vi "FPGA Main.vi"   [LabVIEW 2021]
uses:
  <vilib>/Platform/TimedLoop/XDataNode/timing_clust.ctl
  <vilib>/Platform/TimedLoop/XDataNode/nitl_modes.ctl
  <vilib>/Platform/TimedLoop/XDataNode/wakeup.ctl
  <vilib>/rvi/Emulation/niFpgaGetClockAttributes.vi
  <vilib>/rvi/Emulation/niFpgaSctlEmulationGetInTimedLoop.vi
  <vilib>/rvi/Emulation/niFpgaEmulationReportErrorSimple.vi
  <vilib>/rvi/DataTransferAndStorage/Container/Common/niFpgaContainerGetUniqueNameForEmu.vi
  <vilib>/rvi/DataTransferAndStorage/Container/Common/niFpgaContainerSetEmuInfo.vi
  <vilib>/rvi/eio/common/nirviEmuReportErrorAndStop.vi
  <vilib>/rvi/interface/RandomDataEmulation/niFpgaRandomDataHandleErrors.vi
  <vilib>/rvi/DataTransferAndStorage/Container/Common/niFpgaContainerExecOnDevCompGetState.vi
  <vilib>/rvi/Emulation/niFpgaEmulationIsFPGAContextNoSignature.vi
  <vilib>/rvi/errors/niFpgaSetErrorForExecOnDevCompSimple.vi
  <vilib>/rvi/FIFO/Fifo_Resource/nirvififoEmulationSetSize.vi
  <vilib>/rvi/FIFO/Fifo_Resource/nirviFifoEmulationQueueMgr.vi
  <instcachedir>/0/nirviFifoEmulationQueueMgr_E5CAEC123FF24DC58D834DCA3CDAA9B5.lvgen/nirviFifoEmulationQueueMgr_E5CAEC123FF24DC58D834DCA3CDAA9B5_002.vi
  <vilib>/rvi/FIFO/Fifo_Resource/nirvififoEmulationDetermineInputValidOut.vi
  <vilib>/rvi/FIFO/Fifo_Resource/nirvififoEmulationCreateLock.vi
  <vilib>/rvi/Emulation/niFpgaProcessEmulError.vi
  <vilib>/rvi/FIFO/Fifo_Resource/nirvififoEmulationObtainLock.vi
  <vilib>/rvi/FIFO/Fifo_Resource/nirvififoEmulationReleaseLock.vi
  <vilib>/rvi/occurrence/nirviWaitOnOccurrenceBase.vi
  <vilib>/rvi/errors/nirviReportUnexpectedCaseInternalError.vi
  <vilib>/rvi/errors/nirviReportUnexpectedCaseInternalError (U32).vi
  <vilib>/Utility/error.llb/Clear Errors.vi
  <vilib>/rvi/Emulation/niFpgaCriticalErrorInLSC.vi
  <vilib>/rvi/eio/common/nirviEmuTemplateMethod_errors.vi
  <vilib>/Platform/TimedLoop/XDataNode/XDataNode.xnode
  <vilib>/rvi/LocalResourceManager/LocalResourceManager.xnode
  <vilib>/rvi/DataTransferAndStorage/Container/XNode/niFpgaContainer.xnode
  <vilib>/rvi/interface/RandomDataEmulation/nirviRandomDataFpgaReadWriteTemplate.vi
  <vilib>/rvi/FIFO/Fifo_Resource/niFpgaFifoEmulationRefIn.vi
  <vilib>/eio/EIONode/EIONode.xnode
  <vilib>/Platform/TimedLoop/XDataNode/XDNodeRunTimeDep.lvlib
types:
  T1 = typedef "XDNodeRunTimeDep.lvlib/timing_clust.ctl" = cluster{"Expected End [f-1]":u64, "Actual End [f-1]":u64, "Finished Late? [f-1]":bool, "Expected End [i-1]":u64, "Actual End [i-1]":u64, "Finished Late? [i-1]":bool, "Expected Start [i]":u64, "Actual Start [i]":u64, "Expected Start [f]":u64, "Actual Start [f]":u64, "Source Name":string, "Structure Name":string, "Period":i64, "Deadline":i64, "Offset":i64, "Start":i64, "Priority":i32, "Timeout":i32, "Mode":T2, "Wakeup Reason":T3, "Error":errorcluster, "Source Type":string, "Secondary Source Type":string, "Global End Time":u64, "Global Start Time":u64, "Frame Duration":u64, "Iteration Duration":u64, "Assigned CPU":i32, "I/O Scan Engine Mode":u32}
  T2 = typedef "XDNodeRunTimeDep.lvlib/nitl_modes.ctl" = enum32{"No Change", "Process missed periods, maintain original phase", "Discard missed periods, maintain original phase", "Process missed periods, ignore original phase", "Discard missed periods, ignore original phase"}
  T3 = typedef "XDNodeRunTimeDep.lvlib/wakeup.ctl" = enum32{"Normal", "Aborted", "Asynchronous wakeup", "Timing source error", "Timed loop error", "Timeout"}
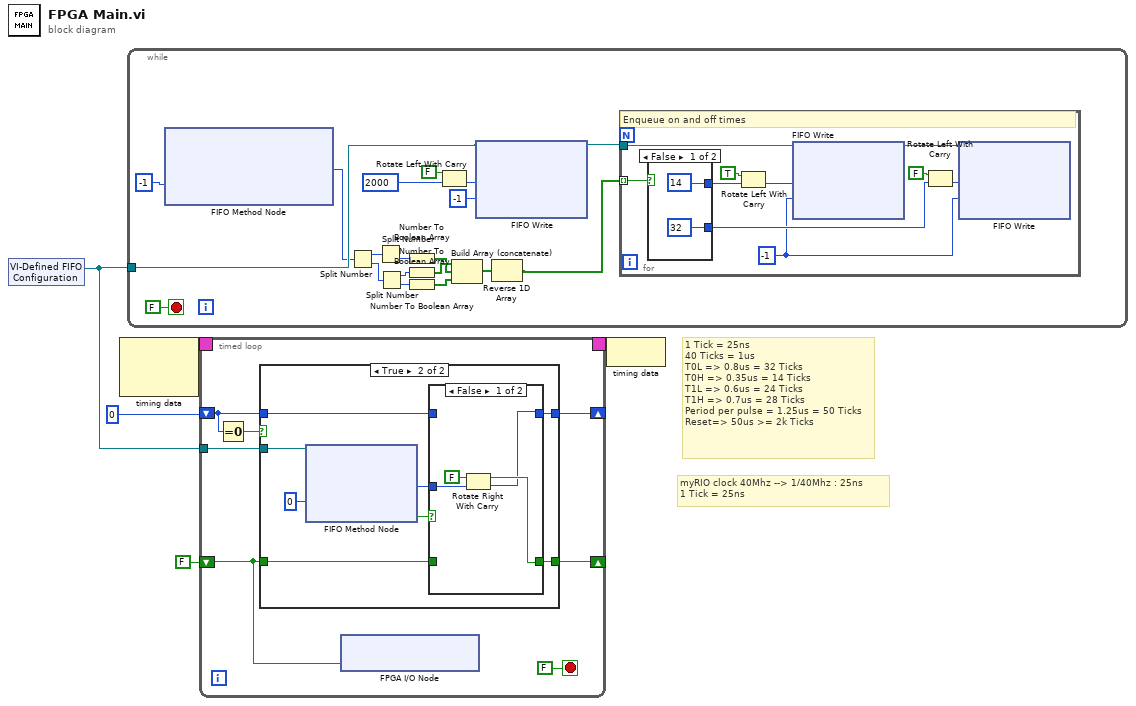
[diagram p0: block diagram]
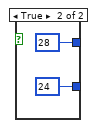
[diagram p2: hidden frame]
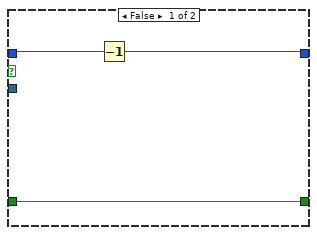
[diagram p3: hidden frame]
diagram:
  # "myRIO clock 40Mhz --> 1/40Mhz : 25ns\n1 Tick = 25ns"
  # "1 Tick = 25ns\n40 Ticks = 1us\nT0L => 0.8us = 32 Ticks \nT0H => 0.35us = 14 Ticks\nT1L => 0.6us = 24 Ticks \nT1H => 0.7us = 28 Ticks\nPeriod per pulse = 1.25us = 50 Ticks\nReset=> 50us >= 2k Ticks"
  n1 = xnode "VI-Defined FIFO Configuration"() -> ("FIFO Out"=w2:refnum<k21>)
  n2 = node-c288() -> (w5:T1)  [unwired: 2 in]
  n3 = while {
    tunnel: w2 -> [w22]
    stop <- FALSE stop-if-true
    n4 = xnode ("FIFO Method Node")("Timeout"=-1) -> ("Element"=w12:u32)  [unwired: 1 in, 2 out]
    n5 = Split Number(x=w12) -> (hi(x)=w21:u16, lo(x)=w20:u16)
    n6 = Split Number(x=w21) -> (lo(x)=w19:u8)  [unwired: 1 out]
    n7 = Split Number(x=w20) -> (hi(x)=w18:u8, lo(x)=w17:u8)
    n8 = Number To Boolean Array(number=w19) -> (Boolean array=w15:bool[])
    n9 = Number To Boolean Array(number=w18) -> (Boolean array=w16:bool[])
    n10 = Number To Boolean Array(number=w17) -> (Boolean array=w14:bool[])
    n11 = Rotate Left With Carry(2:u16 2000, 3:FALSE ("carry")) -> (0:w6:u16)  [unwired: 1 out]
    n12 = Build Array (concatenate)(w16, w15, w14) -> (w13:bool[])
    n13 = xnode ("FIFO Write")("Element"=w6, "Timeout"=-1, "FIFO In"=w22) -> ("FIFO Out"=w7:refnum<k21>)  [unwired: 1 out]
    n14 = Reverse 1D Array(array=w13) -> (reversed array=w11:bool[])
    n15 = for {
      tunnel: w7 -> [w34]
      tunnel: w11 -> [w25] mode=indexing
      w26 = -1 ("Timeout")
      # "Enqueue on and off times"
      n16 = case shown="False" w25 {
        tunnel: [u16 14 u16 28] -> w32
        tunnel: [u16 32 u16 24] -> w29
        frame False {
        }
        frame True {
        }
      }
      n17 = Rotate Left With Carry(2:w32, 3:TRUE ("carry")) -> (0:w31:u16)  [unwired: 1 out]
      n18 = xnode ("FIFO Write")("Element"=w31, "Timeout"=w26, "FIFO In"=w34) -> ("FIFO Out"=w33:refnum<k21>)  [unwired: 1 out]
      n19 = Rotate Left With Carry(2:w29, 3:FALSE ("carry")) -> (0:w27:u16)  [unwired: 1 out]
      n20 = xnode ("FIFO Write")("Element"=w27, "Timeout"=w26, "FIFO In"=w33) -> ()  [unwired: 2 out]
    }
  }
  n21 = timed-loop {
    timing: w5 -> [_]
    timing-out: [_] -> w4
    shift-right: [w44] -> _
    shift-left: FALSE -> [w43]
    tunnel: w2 -> [w42]
    shift-right: [w39] -> _
    shift-left: u16 0 ("Timeout") -> [w40]
    stop <- FALSE stop-if-true
    n22 = Equal To 0?(x=w40) -> (x = 0?=w41:bool)
    n23 = case shown="True" w41 {
      tunnel: [w46 w56] -> w44
      tunnel: w43 -> [w46 w55]
      tunnel: w42 -> [_ w54]
      tunnel: w40 -> [w48 w49]
      tunnel: [w47 w50] -> w39
      frame False {
        n24 = Decrement(x=w48) -> (x-1=w47:u16)
      }
      frame True {
        n25 = xnode ("FIFO Method Node")("Timeout"=0, "FIFO In"=w54) -> ("Element"=w51:u16, "Timed Out?"=w52:bool)  [unwired: 1 out]
        n26 = case shown="False" w52 {
          tunnel: [w58 w62] -> w56
          tunnel: w55 -> [_ w62]
          tunnel: w51 -> [w60 _]
          tunnel: [w57 w61] -> w50
          tunnel: w49 -> [_ w61]
          frame False {
            n27 = Rotate Right With Carry(2:w60, 3:FALSE ("carry")) -> (0:w57:u16, 1:w58:bool)
          }
          frame True {
          }
        }
      }
    }
    n28 = xnode "FPGA I/O Node"("ConnectorC/DIO7"=w43) -> ()  [unwired: 1 in, 1 out]
  }
  n29 = node-c288(w4) -> ()
